vi "프로퍼티노드_인보크노드 실습.vi"() -> ()   [LabVIEW 2020]
panel:
  in  "탭 컨트롤":enum32{"페이지 1", "페이지 2"}(tab)
  out "웨이브폼 차트":dbl(graph)
  out "값":dbl
  out "숫자형 3":dbl
  out "숫자형 2":dbl
  in  "숫자형":dbl
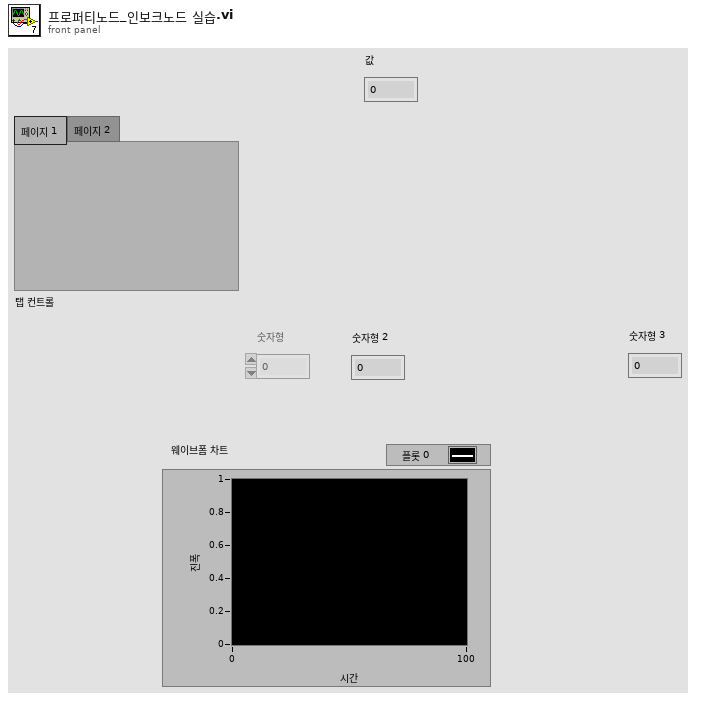
[diagram p1: front panel]
types:
  T1 = enum8{"Enabled", "Disabled", "Disabled and Grayed Out"}
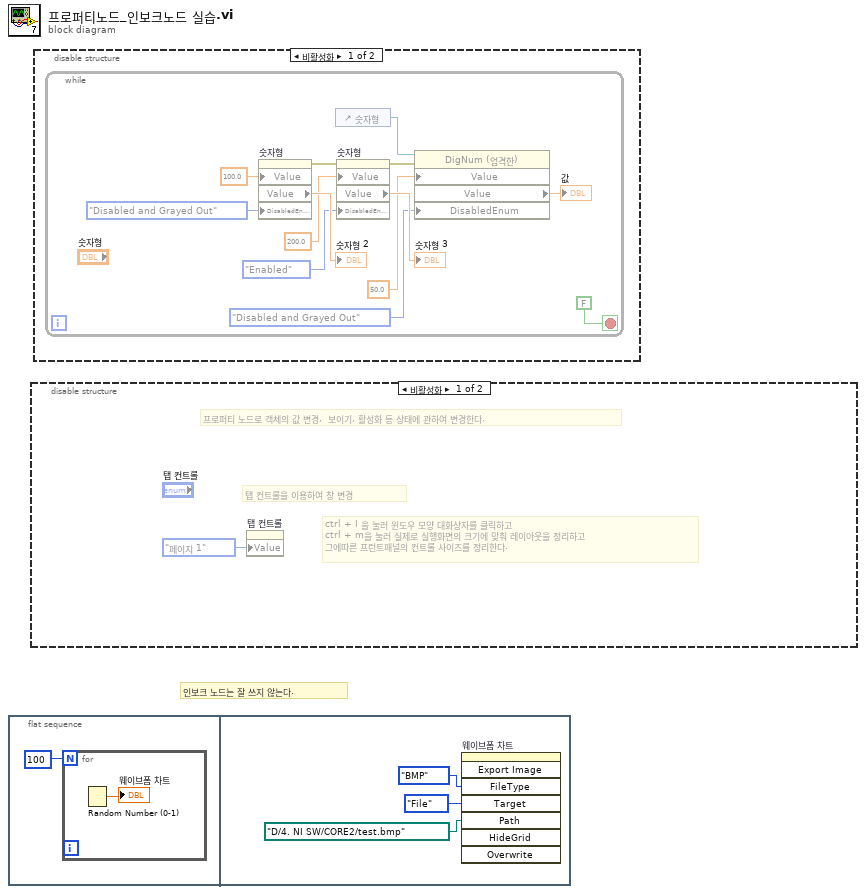
[diagram p0: block diagram]
diagram:
  # "인보크 노드는 잘 쓰지 않는다."
  n1 = flat-sequence {
    frame #0 {
      n2 = for {
        N: 100 -> [_]
        n3 = Random Number (0-1)() -> (number: 0 to 1=→"웨이브폼 차트":dbl)
      }
    }
    frame #1 {
      n4 = invoke on="웨이브폼 차트" class="WFChart (엄격한)" method="Export Image"("FileType"=enum32{"BMP", "EPS", "EMF", "PICT"}."BMP" ("파일 타입"), "Target"=enum32{"File", "Clipboard"}."File" ("타겟"), "Path"=path "D:/4. NI SW/CORE2/test.bmp" ("경로")) -> ()  [unwired: 5 in, 8 out]
    }
  }
  n5 = disable-structure shown="비활성화" {
    frame Disabled {
      # "ctrl + I 을 눌러 윈도우 모양 대화상자를 클릭하고\nctrl + m을 눌러 실제로 실행화면의 크기에 맞춰 레이아웃을 정리하고\n그에따른 프런트패널의 컨트롤 사이즈를 정리한다."
      # "탭 컨트롤을 이용하여 창 변경"
      # "프로퍼티 노드로 객체의 값 변경,  보이기, 활성화 등 상태에 관하여 변경한다."
      n6 = property on="탭 컨트롤" class="TabCtl (엄격한)"("Value"=enum32{"페이지 1", "페이지 2"}."페이지 1" ("탭 컨트롤")) -> ()  [unwired: 2 in, 2 out]
    }
    frame Enabled {
    }
  }
  n7 = disable-structure shown="비활성화" {
    frame Disabled {
      n8 = while {
        stop <- FALSE stop-if-true
        n9 = property on="숫자형" class="DigNum (엄격한)"("Value"=100.0 ("숫자형"), "DisabledEnum"=T1."Disabled and Grayed Out" ("비활성화")) -> (error out=w13:errorcluster, "Value"=→"숫자형 2":dbl)  [unwired: 2 in, 1 out]
        n10 = control-ref of="숫자형"() -> (w12:refnum<vi>)
        n11 = property on="숫자형" class="DigNum (엄격한)"(error in=w13, "Value"=200.0 ("숫자형"), "DisabledEnum"=T1."Enabled" ("비활성화")) -> (error out=w8:errorcluster, "Value"=→"숫자형 3":dbl)  [unwired: 1 in, 1 out]
        n12 = property class="DigNum (엄격한)"(reference=w12, error in=w8, "Value"=50.0 ("값"), "DisabledEnum"=T1."Disabled and Grayed Out" ("비활성화")) -> ("Value"=→"값":dbl)  [unwired: 2 out]
      }
    }
    frame Enabled {
    }
  }
